vi "UIRef.vi"(8 "error in":errorcluster, 11 "fixed channel editor in":refnum<class "WaveformAcq editor node.lvclass">) -> (0 "error out":errorcluster, 2 "VI refnum":refnum<vi>, 3 "fixed channel editor out":refnum<class "WaveformAcq editor node.lvclass">)   [LabVIEW 2017, in "WaveformAcq editor node.lvclass"]
uses:
  WaveformAcq editor node.lvclass
  config UI.vi
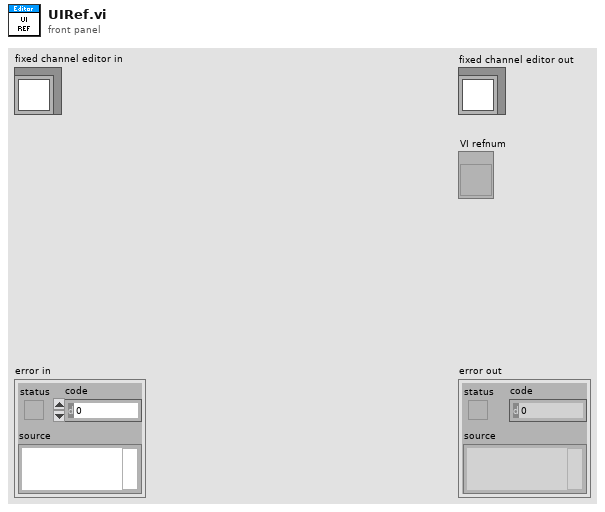
[diagram p1: front panel]
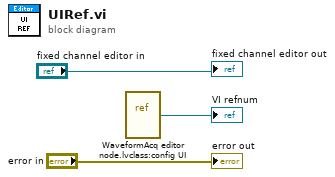
[diagram p0: block diagram]
diagram:
  n1 = vi-ref "WaveformAcq editor node.lvclass:config UI.vi"() -> (→"VI refnum":refnum<vi>)
  "error out" <- "error in"
  "fixed channel editor out" <- "fixed channel editor in"
